vi "SaveArm.vi"(8 "Error In":errorcluster, 11 ".NET Refnum in":refnum<k24>) -> (0 "Error Out":errorcluster, 3 "LEAParm":T1)   [LabVIEW 2017, in "LeapMotion.lvlib"]
uses:
  LeapMotion.lvlib
  C:/Users/snordinh/Desktop/LEAP/LEAP-sign-language-test/LeapMotion/Dynamic Libraries/LeapCSharp.NET4.5.dll
  Dynamic Libraries/LeapCSharp.NET4.5.dll
  TypeDefs/LEAParm.ctl
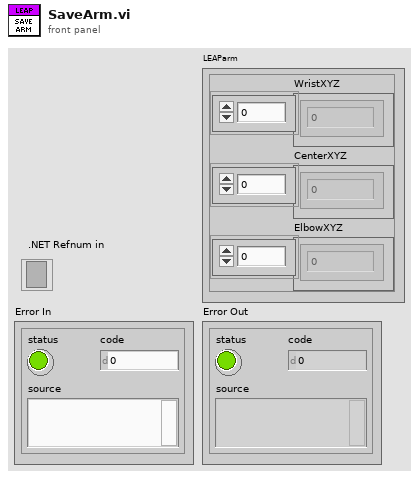
[diagram p1: front panel]
types:
  T1 = typedef "LeapMotion.lvlib/LEAParm.ctl" = cluster{"WristXYZ":sgl[], "CenterXYZ":sgl[], "ElbowXYZ":sgl[]}
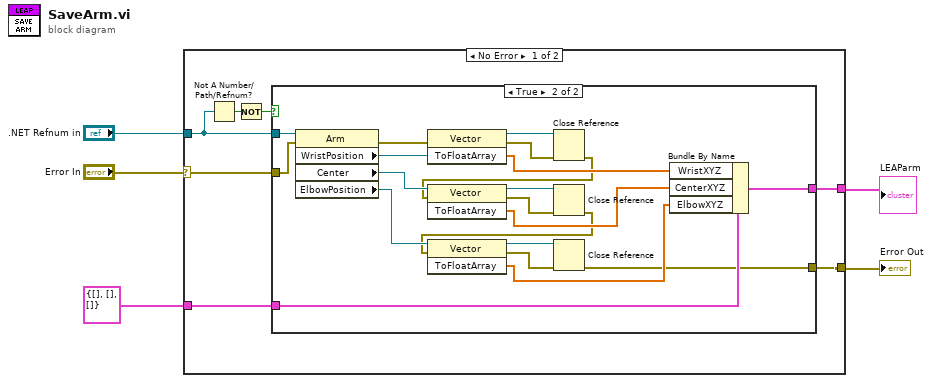
[diagram p0: block diagram]
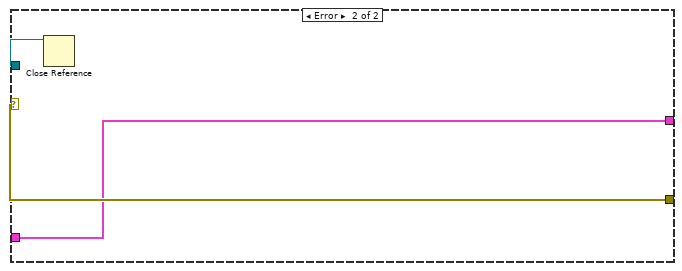
[diagram p3: hidden frame]
diagram:
  n1 = case shown="No Error" "Error In" {
    selector: "Error In" -> [w9 w37]
    tunnel: ".NET Refnum in" -> [w11 w35]
    tunnel: [w8 w36] -> w4
    tunnel: [w7 w37] -> w1
    tunnel: T1 {"WristXYZ"=[], "CenterXYZ"=[], "ElbowXYZ"=[]} -> [w6 w36]
    frame No Error {
      n2 = Not A Number/Path/Refnum?(number/path/refnum=w11) -> (NaN/Path/Refnum?=w12:bool)
      n3 = Not(x=w12) -> (.not. x?=w10:bool)
      n4 = case shown="True" w10 {
        tunnel: w11 -> [_ w34]
        tunnel: w9 -> [w14 w26]
        tunnel: [w13 w25] -> w8
        tunnel: [w14 w15] -> w7
        tunnel: w6 -> [w13 w24]
        frame False {
        }
        frame True {
          n5 = property class="Arm"(reference=w34, error in=w26) -> (error out=w30:errorcluster, "WristPosition"=w33:refnum<k24>, "Center"=w32:refnum<k24>, "ElbowPosition"=w31:refnum<k24>)  [unwired: 1 out]
          n6 = invoke class="Vector" method="ToFloatArray"(reference=w33, error in=w30) -> (reference out=w21:refnum<k24>, error out=w20:errorcluster, "ToFloatArray"=w29:sgl[])  [unwired: 1 in]
          n7 = Close Reference(reference=w21, error in (no error)=w20) -> (error out=w19:errorcluster)
          n8 = invoke class="Vector" method="ToFloatArray"(reference=w32, error in=w19) -> (reference out=w22:refnum<k24>, error out=w18:errorcluster, "ToFloatArray"=w28:sgl[])  [unwired: 1 in]
          n9 = Close Reference(reference=w22, error in (no error)=w18) -> (error out=w17:errorcluster)
          n10 = invoke class="Vector" method="ToFloatArray"(reference=w31, error in=w17) -> (reference out=w23:refnum<k24>, error out=w16:errorcluster, "ToFloatArray"=w27:sgl[])  [unwired: 1 in]
          n11 = Close Reference(reference=w23, error in (no error)=w16) -> (error out=w15:errorcluster)
          n12 = Bundle By Name(cluster=w24, "WristXYZ"=w29, "CenterXYZ"=w28, "ElbowXYZ"=w27) -> (w25:T1)
        }
      }
    }
    frame Error {
      n13 = Close Reference(reference=w35) -> ()  [unwired: 1 in, 1 out]
    }
  }
  "LEAParm" <- w4
  "Error Out" <- w1
